vi "Read Adjacent Containers.vi"(7 "Exclude Source":refnum<class "Message Enqueuer.lvclass">, 8 "error in (no error)":errorcluster, 11 "Sample Line in":refnum<class "Sample Line.lvclass">) -> (0 "error out":errorcluster, 2 "Adjacent Containers":refnum<class "Message Enqueuer.lvclass">[](array[class]), 3 "Sample Line out":refnum<class "Sample Line.lvclass">)   [LabVIEW 2015, in "cRIO-Carbondioxide.lvlib" / "CO2-Actor.lvlib" / "Sample Line.lvclass"]
uses:
  Sample Line.lvclass
  <vilib>/ActorFramework/Message Enqueuer/Message Enqueuer.lvclass
  CO2 Actor/CO2 Actor.lvclass
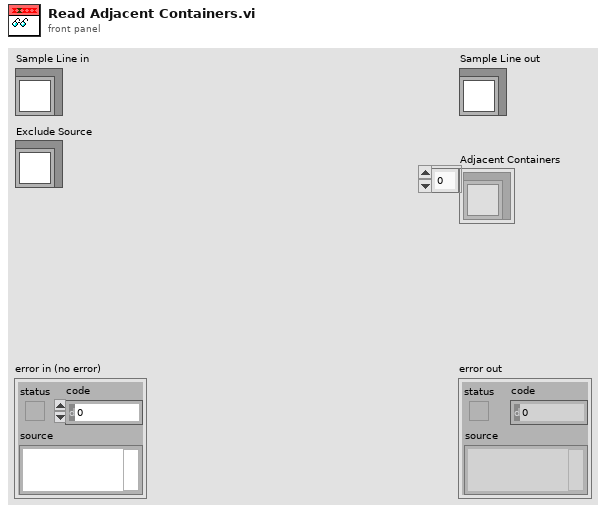
[diagram p1: front panel]
types:
  T1 = typedef "Dedicated Enqueuers.ctl" = cluster{"Freezers":cluster{"Syringe":refnum<class "Message Enqueuer.lvclass">, "Tank 1":refnum<class "Message Enqueuer.lvclass">, "Tank 2":refnum<class "Message Enqueuer.lvclass">, "Tank 3":refnum<class "Message Enqueuer.lvclass">, "Tank 4":refnum<class "Message Enqueuer.lvclass">}, "Heaters":cluster{"Syringe":refnum<class "Message Enqueuer.lvclass">, "Piston":refnum<class "Message Enqueuer.lvclass">}, "Blowers":cluster{"Tank 1":refnum<class "Message Enqueuer.lvclass">, "Tank 2":refnum<class "Message Enqueuer.lvclass">, "Tank 3":refnum<class "Message Enqueuer.lvclass">, "Tank 4":refnum<class "Message Enqueuer.lvclass">, "Syringe":refnum<class "Message Enqueuer.lvclass">}, "Sample Line":refnum<class "Message Enqueuer.lvclass">, "Storage Line":refnum<class "Message Enqueuer.lvclass">, "Transfer Line":refnum<class "Message Enqueuer.lvclass">, "Syringe Stepper":refnum<class "Message Enqueuer.lvclass">, "Syringe Line":refnum<class "Message Enqueuer.lvclass">, "Capillary Line":refnum<class "Message Enqueuer.lvclass">, "Preparation Line":refnum<class "Message Enqueuer.lvclass">, "Turbo":refnum<class "Message Enqueuer.lvclass">, "Vacuum":refnum<class "Message Enqueuer.lvclass">, "He Line":refnum<class "Message Enqueuer.lvclass">, "Cylinder":refnum<class "Message Enqueuer.lvclass">}
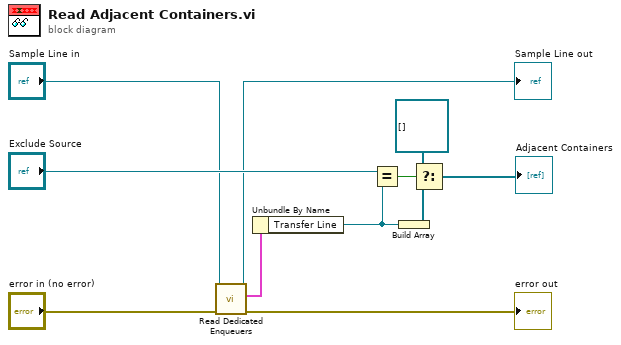
[diagram p0: block diagram]
diagram:
  n1 = call "Read Dedicated Enqueuers.vi"("error in (no error)"="error in (no error)", "CO2 Actor in"="Sample Line in") -> ("error out"=→"error out":errorcluster, "Dedicated Enqueuers"=w11:T1, "CO2 Actor out"=→"Sample Line out":refnum<class "Sample Line.lvclass">)  [unwired: 6 in, 1 out]
  n2 = Unbundle By Name(w11) -> ("Transfer Line"=w3:refnum<class "Message Enqueuer.lvclass">)
  n3 = Equal?(x="Exclude Source", y=w3) -> (x = y?=w8:bool)
  n4 = Build Array(w3) -> (w7:refnum<class "Message Enqueuer.lvclass">[])
  n5 = Select(t=refnum<class "Message Enqueuer.lvclass">[] [], s=w8, f=w7) -> (s? t:f=→"Adjacent Containers":refnum<class "Message Enqueuer.lvclass">[])
